vi "EvaluateGenericBooleanTriggerExpression.vi"(8 "error in (no error)":errorcluster, 9 "expression":string, 10 "all conditions":T1[](array[typedef])=[{"Condition"={"Source"="", "Type"="", "Operator"="", "CompareTo"="", "DwellSeconds"=0.0}, "LatchValue"="", "LatchTime"=timestamp(0 s since 1904-01-01)}, {"Condition"={"Source"="", "Type"="", "Operator"="", "CompareTo"="", "DwellSeconds"=0.0}, "LatchValue"="", "LatchTime"=timestamp(0 s since 1904-01-01)}], 11 "map":T3) -> (0 "error out":errorcluster, 2 "all conditions out":T1[](array[typedef]), 3 "trigger":bool, 4 "triggered conditions":T1[](array[typedef]))   [LabVIEW 2017, in "Trigger.lvlib"]
uses:
  <vilib>/addons/InsightCM/Devices/Shared/Common/Trigger/Trigger.lvlib
  <vilib>/addons/InsightCM/Devices/Shared/Common/Trigger/controls/TriggerCondition.ctl
  <vilib>/addons/InsightCM/MessageBus/Base/controls/Condition.ctl
  <vilib>/addons/PointValueMap/controls/PointMap.ctl
  <vilib>/addons/InsightCM/Utilities/ExpressionEvaluator/ExpressionEvaluator.lvlib
  <vilib>/addons/PointValueMap/PointValueMap.lvlib
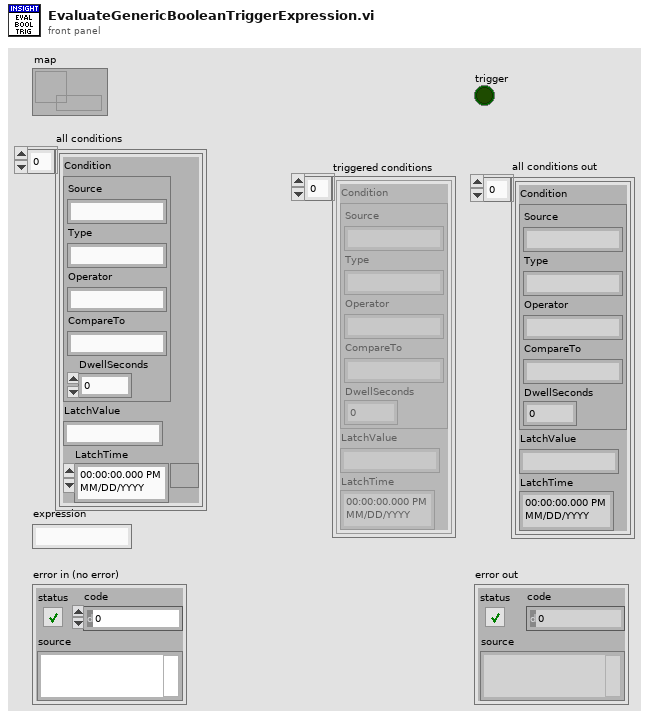
[diagram p1: front panel]
types:
  T1 = typedef "Trigger.lvlib/TriggerCondition.ctl" = cluster{"Condition":T2, "LatchValue":string, "LatchTime":timestamp}
  T2 = typedef "Condition.ctl" = cluster{"Source":string, "Type":string, "Operator":string, "CompareTo":string, "DwellSeconds":dbl}
  T3 = typedef "PointValueMap.lvlib/PointMap.ctl" = refnum<data-value>
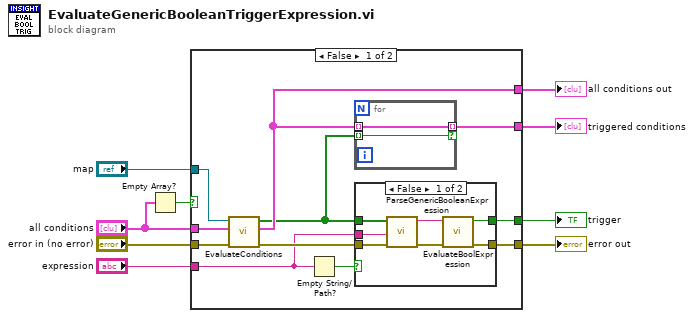
[diagram p0: block diagram]
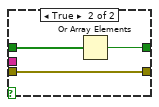
[diagram p2: hidden frame]
diagram:
  n1 = Empty Array?(array="all conditions") -> (empty?=w2:bool)
  n2 = case shown="False" w2 {
    tunnel: "error in (no error)" -> [w20 w33]
    tunnel: "map" -> [w19 _]
    tunnel: [w17 w33] -> w7
    tunnel: [w16 _] -> w6
    tunnel: "expression" -> [w15 _]
    tunnel: [w12 _] -> w4
    tunnel: "all conditions" -> [w14 _]
    tunnel: [w11 _] -> w1
    frame False {
      n3 = call <vilib>:"EvaluateConditions.vi"("error in (no error)"=w20, "conditions in"=w14, "map"=w19) -> ("error out"=w18:errorcluster, "conditions out"=w12:T1[], "trigger"=w10:bool[])  [unwired: 5 in, 1 out]
      n4 = Empty String/Path?(string/path=w15) -> (empty?=w13:bool)
      n5 = for {
        tunnel: w12 -> [w22] mode=indexing
        tunnel: [w22] -> w11 mode=indexing if=w21
        tunnel: w10 -> [w21] mode=indexing
      }
      n6 = case shown="False" w13 {
        tunnel: w18 -> [w29 w32]
        tunnel: w10 -> [w28 w31]
        tunnel: [w26 w32] -> w17
        tunnel: [w25 w30] -> w16
        tunnel: w15 -> [w23 _]
        frame False {
          n7 = call <vilib>:"ParseGenericBooleanExpression.vi"("error in (no error)"=w29, "ConditionExpression"=w23, "bool trigger array"=w28) -> ("error out"=w27:errorcluster, "expression"=w24:string)  [unwired: 7 in]
          n8 = call <vilib>:"EvaluateBoolExpression.vi"("error in (no error)"=w27, "infix expression"=w24) -> ("error out"=w26:errorcluster, "result"=w25:bool)  [unwired: 8 in]
        }
        frame True {
          n9 = Or Array Elements(Boolean array=w31) -> (logical OR=w30:bool)
        }
      }
    }
    frame True {
    }
  }
  "error out" <- w7
  "trigger" <- w6
  "all conditions out" <- w4
  "triggered conditions" <- w1
